vi "54 Occurences and more.vi"() -> ()   [LabVIEW 2019]
uses:
  _Subs/OpenDiagram/Open_XControl.xctl
panel:
  in  "OpenDiag":refnum<vi>(xcontrol)
  out "Semaphore loop":i32
  out "Total Fired":u8
  out "Total Occurrences Fired":u8
  out "Current Loop 1 Iteration":i32
  in  "Stop":bool
  # "04 Occurences and more\nThis code shows how occurences and semaphores work  \n\nInstructions:\n1. Hit the Run arrow and see the loop interations change"
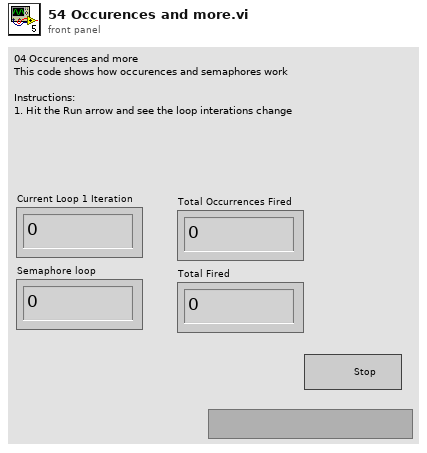
[diagram p1: front panel]
types:
  T1 = typedef "Semaphore RefNum" = refnum<k1>
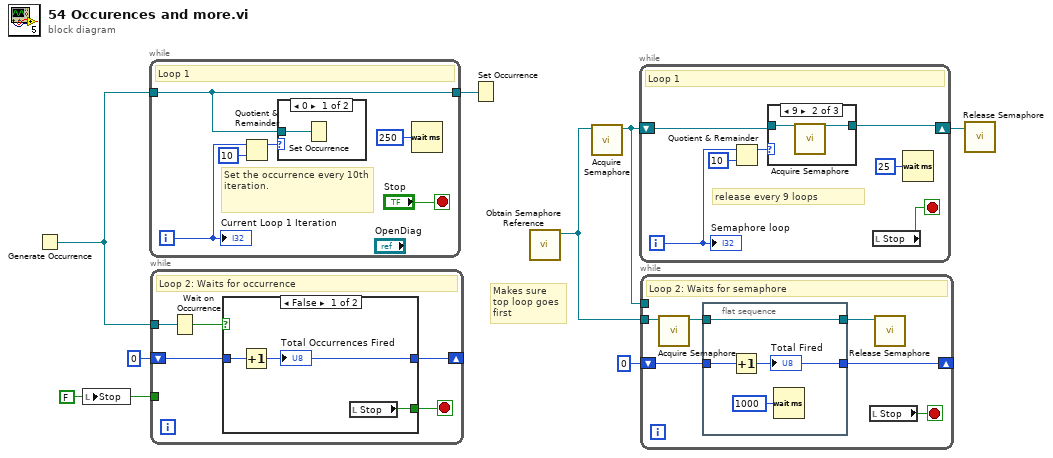
[diagram p0: block diagram]
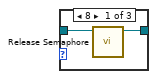
[diagram p2: hidden frame]
diagram:
  w5 = FALSE ("Loop Stop")
  # "Makes sure\ntop loop goes\nfirst"
  n1 = Generate Occurrence() -> (w8:refnum<k4>)
  n2 = local write "Stop"(w5) -> ()
  n3 = while {
    tunnel: w8 -> [w12]
    tunnel: [w12] -> w7
    i -> [w9]
    stop <- "Stop" stop-if-true
    # "Set the occurrence every 10th iteration."
    # "Loop 1"
    n4 = Quotient & Remainder(x=w9, y=10) -> (x-y*floor(x/y)=w13:i32)  [unwired: 1 out]
    n5 = case shown="0" w13 {
      tunnel: w12 -> [w15 _]
      frame 0 {
        n6 = Set Occurrence(w15) -> ()
      }
      frame Default {
      }
    }
    n7 = Wait (ms)(milliseconds to wait=u32 250) -> ()  [unwired: 1 out]
    "Current Loop 1 Iteration" <- w9
  }
  n8 = while {
    tunnel: w8 -> [w20]
    shift-right: [w17] -> _
    shift-left: u8 0 -> [w18]
    tunnel: w5 -> [_]
    stop <- w16 stop-if-true
    # "Loop 2: Waits for occurrence"
    n9 = Wait on Occurrence(2:w20) -> (0:w19:bool)  [unwired: 2 in]
    n10 = case shown="False" w19 {
      tunnel: [w21 _] -> w16
      tunnel: w18 -> [w23 w24]
      tunnel: [w22 w24] -> w17
      frame False {
        n11 = Increment(x=w23) -> (x+1=w22:u8)
        "Total Occurrences Fired" <- w22
        n12 = local read "Stop"() -> (w21:bool)
      }
      frame True {
      }
    }
  }
  n13 = Set Occurrence(w7) -> ()
  n14 = call <vilib>:"Obtain Semaphore Reference.vi"() -> ("semaphore"=w2:T1)  [unwired: 5 in, 2 out]
  n15 = call <vilib>:"Acquire Semaphore.vi"("semaphore"=w2) -> ("semaphore out"=w1:T1)  [unwired: 4 in, 2 out]
  n16 = while {
    shift-right: [w25] -> w3
    shift-left: w1 -> [w26]
    i -> [w28]
    stop <- w27 stop-if-true
    # "release every 9 loops"
    # "Loop 1"
    n17 = Quotient & Remainder(x=w28, y=10) -> (x-y*floor(x/y)=w30:i32)  [unwired: 1 out]
    n18 = case shown="9" w30 {
      tunnel: w26 -> [w33 w35 w36]
      tunnel: [w32 w34 w36] -> w25
      frame 8 {
        n19 = call <vilib>:"Release Semaphore.vi"("semaphore"=w33) -> ("semaphore out"=w32:T1)  [unwired: 5 in, 1 out]
      }
      frame 9 {
        n20 = call <vilib>:"Acquire Semaphore.vi"("semaphore"=w35) -> ("semaphore out"=w34:T1)  [unwired: 4 in, 2 out]
      }
      frame Default {
      }
    }
    n21 = local read "Stop"() -> (w27:bool)
    n22 = Wait (ms)(milliseconds to wait=u32 25) -> ()  [unwired: 1 out]
    "Semaphore loop" <- w28
  }
  n23 = while {
    shift-right: [w41] -> _
    shift-left: u8 0 -> [w42]
    tunnel: w2 -> [w39]
    tunnel: w1 -> [_]
    stop <- w40 stop-if-true
    # "Loop 2: Waits for semaphore"
    n24 = call <vilib>:"Acquire Semaphore.vi"("semaphore"=w39) -> ("semaphore out"=w37:T1)  [unwired: 4 in, 2 out]
    n25 = flat-sequence {
      tunnel: w42 -> [w46]
      tunnel: [w45] -> w41
      tunnel: [w43] -> w38
      tunnel: w37 -> [w43]
      frame #0 {
        n26 = Increment(x=w46) -> (x+1=w45:u8)
        "Total Fired" <- w45
        n27 = Wait (ms)(milliseconds to wait=u32 1000) -> ()  [unwired: 1 out]
      }
    }
    n28 = local read "Stop"() -> (w40:bool)
    n29 = call <vilib>:"Release Semaphore.vi"("semaphore"=w38) -> ()  [unwired: 5 in, 2 out]
  }
  n30 = call <vilib>:"Release Semaphore.vi"("semaphore"=w3) -> ()  [unwired: 5 in, 2 out]
